vi "FTW-Message-Request-Construct.vi"(8 "error in":errorcluster, 9 "Multipart Message":string[](array[string]), 10 "Frontend Endpoint":refnum<class "FTW-Endpoint.lvclass">) -> (0 "error out":errorcluster, 3 "FTW Incoming Request":refnum<class "FTW-Message-IncomingRequest.lvclass">)   [LabVIEW 2013, in "FTW-Message-IncomingRequest.lvclass"]
uses:
  FTW-Message-IncomingRequest.lvclass
  Endpoint/FTW-Endpoint.lvclass
  FTW-Message-IncomingRequest.lvclass/FTW-Message-IncomingRequest.ctl
panel:
  # "Inputs"
  # "Outputs"
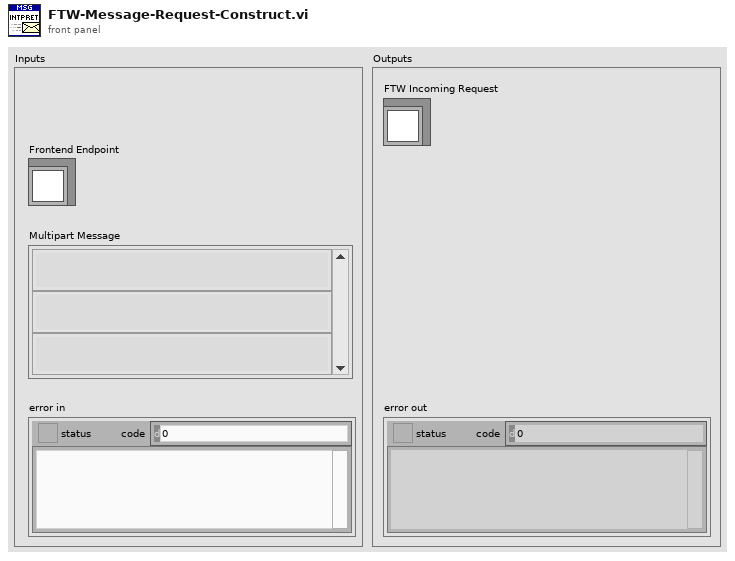
[diagram p1: front panel]
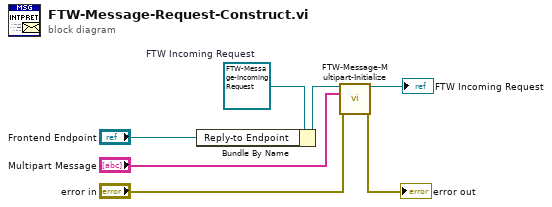
[diagram p0: block diagram]
diagram:
  w3 = refnum<class "FTW-Message-IncomingRequest.lvclass"> refnum  # FTW Incoming Request
  n1 = Bundle By Name(cluster=w3, "Reply-to Endpoint"="Frontend Endpoint") -> (w2:refnum<class "FTW-Message-IncomingRequest.lvclass">)
  n2 = call-dynamic "FTW-Message-Multipart-Initialize.vi"("FTW Message"=w2, "Message Parts"="Multipart Message", "error in"="error in") -> ("FTW Message out"=→"FTW Incoming Request":refnum<class "FTW-Message-IncomingRequest.lvclass">, "error out"=→"error out":errorcluster)  [unwired: 11 in]
